vi "Fix Relocated Connections.vi"(8 "error in (no error)":errorcluster, 10 "Outdated Dependent Modules":cluster{"Old Path":string, "New Path":string}[](array[cluster]), 11 "Routing Channels Ref in":T1 format="%.0x") -> (0 "error out":errorcluster, 3 "Routing Channels Ref out":T1 format="%.0x")   [LabVIEW 2017, in "Routing and Faulting System Explorer.lvlib"]
uses:
  Routing and Faulting System Explorer.lvlib
  <vilib>/NI Veristand/Custom Device API/Custom Device Item Ref.ctl
  Scripting/Routing and Faulting Scripting.lvlib
  <vilib>/NI Veristand/Custom Device API/Custom Device API.lvlib
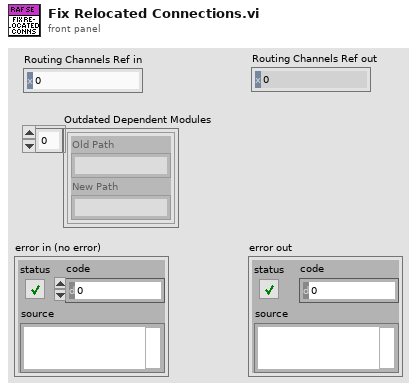
[diagram p1: front panel]
types:
  T1 = typedef "Custom Device API.lvlib/Custom Device Item Ref.ctl" = u64
  T2 = typedef "Routing and Faulting Shared.lvlib/Channel States.ctl" = T3[]
  T3 = typedef "Routing and Faulting Shared.lvlib/Routing State.ctl" = cluster{"Name":string, "Description":string, "Value":i32, "Connection List":T4[]}
  T4 = typedef "Routing and Faulting Shared.lvlib/Connection.ctl" = cluster{"Module":string, "Source":string, "Destination":string}
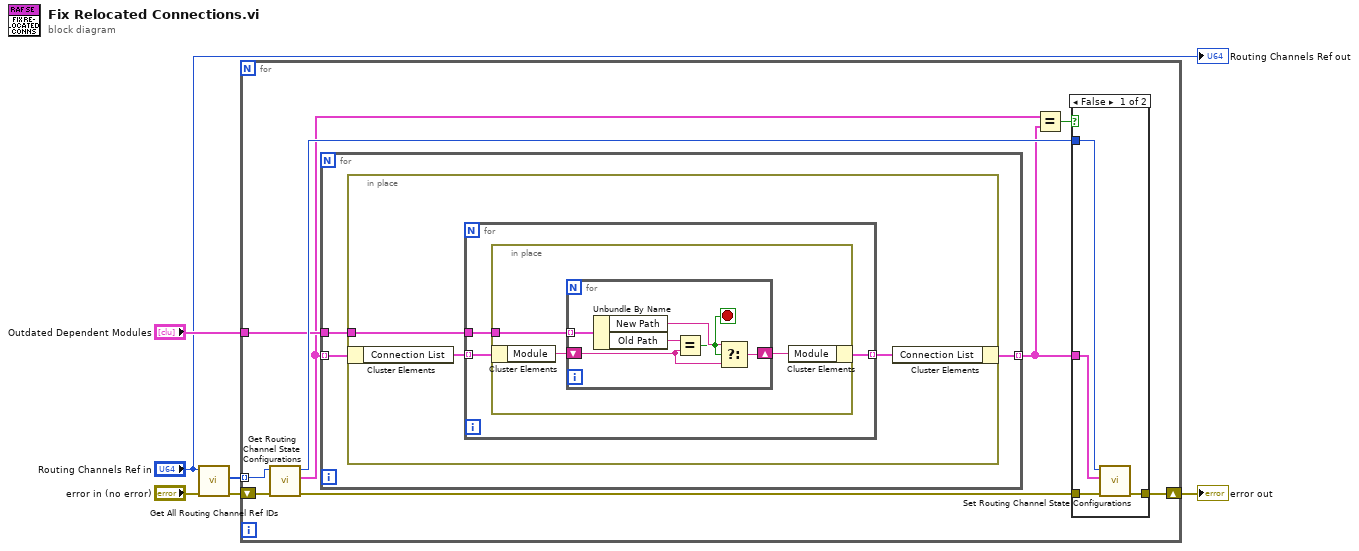
[diagram p0: block diagram]
diagram:
  n1 = call "Get All Routing Channel Ref IDs.vi"("error in (no error)"="error in (no error)", "Routing Channels Ref in"="Routing Channels Ref in") -> ("error out"=w2:errorcluster, "Channel Refs"=w1:T1[])  [unwired: 7 in, 1 out]
  n2 = for {
    tunnel: w1 -> [w12] mode=indexing
    shift-right: [w13] -> w4
    shift-left: w2 -> [w14]
    tunnel: "Outdated Dependent Modules" -> [w10]
    n3 = call "Get Routing Channel State Configurations.vi"("error in (no error)"=w14, "Channel Ref in"=w12) -> ("error out"=w11:errorcluster, "State Configurations"=w7:T2, "Channel Ref out"=w15:T1)  [unwired: 7 in]
    n4 = for {
      tunnel: w7 -> [w23] mode=indexing
      tunnel: [w22] -> w8 mode=indexing
      tunnel: w10 -> [w21]
      n5 = in-place {
        in-place-border: w21 -> [w26]
        n6 = in-place-cluster #1(w23) -> ("Connection List"=w25:T4[])
        n7 = for {
          tunnel: w26 -> [w29]
          tunnel: w25 -> [w28] mode=indexing
          tunnel: [w27] -> w24 mode=indexing
          n8 = in-place {
            in-place-border: w29 -> [w32]
            n9 = in-place-cluster #2(w28) -> ("Module"=w31:string)
            n10 = for {
              tunnel: w32 -> [w38] mode=indexing
              shift-right: [w35] -> w30
              shift-left: w31 -> [w36]
              stop <- w33 stop-if-true
              n11 = Unbundle By Name(w38) -> ("New Path"=w34:string, "Old Path"=w37:string)
              n12 = Equal?(x=w37, y=w36) -> (x = y?=w33:bool)
              n13 = Select(t=w34, s=w33, f=w36) -> (s? t:f=w35:string)
            }
            n14 = in-place-cluster #2("Module"=w30) -> (w27:T4)
          }
        }
        n15 = in-place-cluster #1("Connection List"=w24) -> (w22:T3)
      }
    }
    n16 = Equal?(x=w7, y=w8) -> (x = y?=w9:bool)
    n17 = case shown="False" w9 {
      tunnel: w15 -> [w19 _]
      tunnel: [w18 w20] -> w13
      tunnel: w11 -> [w17 w20]
      tunnel: w8 -> [w16 _]
      frame False {
        n18 = call "Set Routing Channel State Configurations.vi"("error in (no error)"=w17, "State Configurations"=w16, "Channel Ref in"=w19) -> ("error out"=w18:errorcluster)  [unwired: 7 in, 1 out]
      }
      frame True {
      }
    }
  }
  "error out" <- w4
  "Routing Channels Ref out" <- "Routing Channels Ref in"
